vi "Read SFTP Refnum.vi"(8 "error in (no error)":errorcluster, 11 "sftp":T2) -> (0 "error out":errorcluster, 2 "LIBSSH2_SFTP*":u64, 3 "session":T1)   [LabVIEW 2017, in "libssh2.lvlib"]
doc: "Read <B>LIBSSH2_SFTP*</B> associated with <B>sftp</B>."
uses:
  libssh2.lvlib
  SFTP Refnum.ctl
  Session Refnum.ctl
  SFTP Refnum Data.ctl
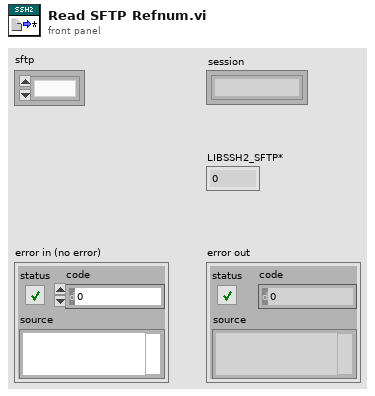
[diagram p1: front panel]
types:
  T1 = typedef "libssh2.lvlib/Session Refnum.ctl" = refnum<k1>
  T2 = typedef "libssh2.lvlib/SFTP Refnum.ctl" = refnum<k1>
  T3 = typedef "libssh2.lvlib/SFTP Refnum Data.ctl" = cluster{"LIBSSH2_SFTP*":u64, "session":T1}
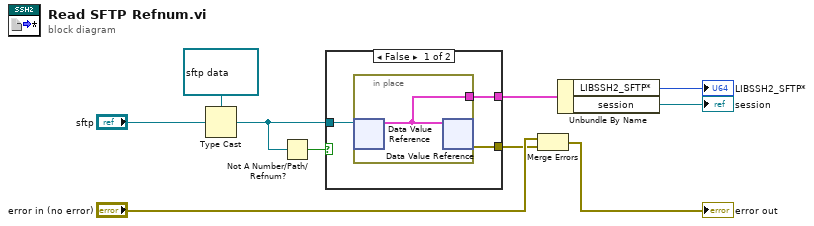
[diagram p0: block diagram]
diagram:
  n1 = Type Cast(type=refnum<data-value> refnum ("data value reference"), x="sftp") -> (*(type *) &x=w4:refnum<data-value>)
  n2 = Not A Number/Path/Refnum?(number/path/refnum=w4) -> (NaN/Path/Refnum?=w3:bool)
  n3 = case shown="False" w3 {
    tunnel: w4 -> [w13 _]
    tunnel: [w12 _] -> w9
    tunnel: [w11 _] -> w5
    frame False {
      n4 = in-place {
        in-place-border: [w14] -> w12
        n5 = in-place-dvr #1(w13) -> (w14:T3)  [unwired: 1 out]
        n6 = in-place-dvr #1(w14) -> (w11:errorcluster)  [unwired: 1 out]
      }
    }
    frame True {
    }
  }
  n7 = Merge Errors("error in (no error)", w5) -> (→"error out":errorcluster)
  n8 = Unbundle By Name(w9) -> ("LIBSSH2_SFTP*"=→"LIBSSH2_SFTP*":u64, "session"=→"session":T1)
